vi "CRYGet LoadFileName.vi"(4 "pattern label":string, 5 "ButtonName":string="OK", 6 "pattern (all files)":string="*.cre", 7 "TitleName":string="Open", 8 "error in":errorcluster, 9 "Category Name":string="cre", 10 "default name":string, 11 "Start path":path) -> (0 "error out":errorcluster, 1 "stripped path":path, 2 "Which Button?":T1(ring), 3 "Path":path)   [LabVIEW 2013]
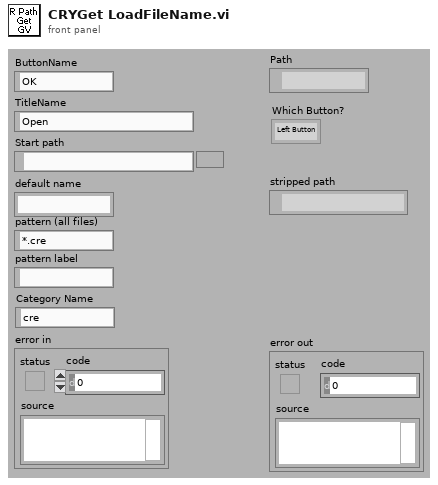
[diagram p1: front panel]
types:
  T1 = enum16{"Left Button", "Center Button", "Right Button", "Window Close"}
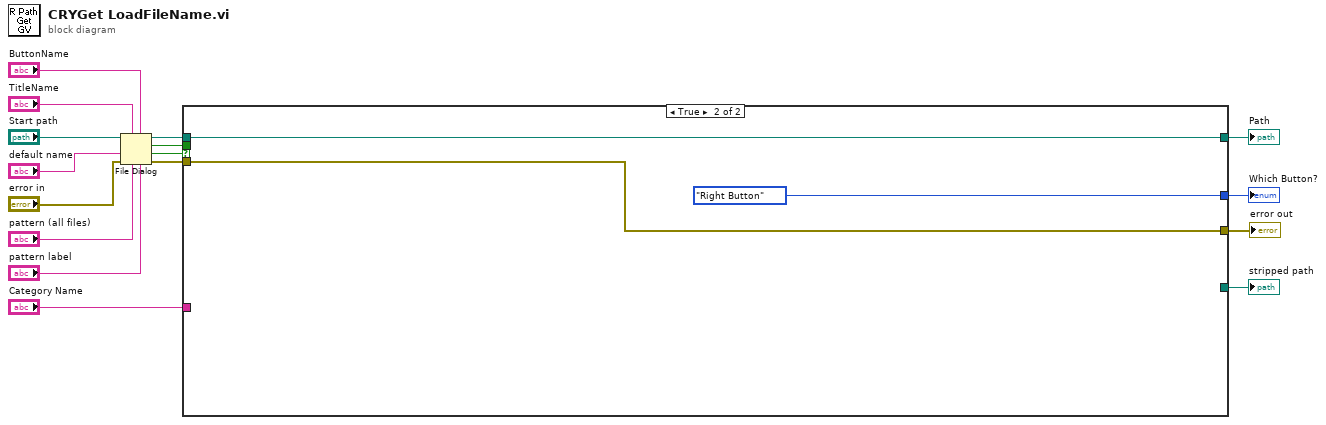
[diagram p0: block diagram]
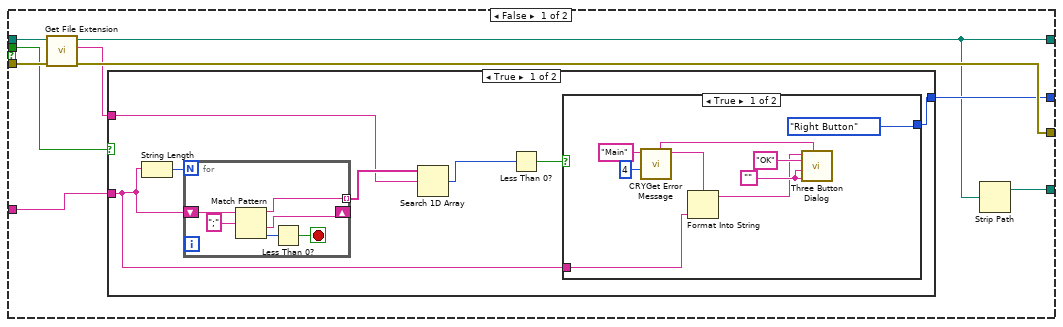
[diagram p2: hidden frame]
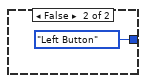
[diagram p3: hidden frame]
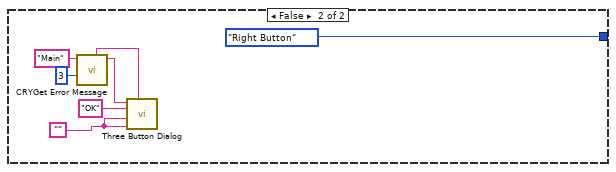
[diagram p4: hidden frame]
diagram:
  n1 = File Dialog(4:"pattern label", 5:"ButtonName", 6:"pattern (all files)", 7:"TitleName", 8:"error in", 9:"default name", 11:"Start path") -> (0:w6:errorcluster, 1:w12:bool, 2:w2:bool, 3:w14:path)
  n2 = case shown="True" w12 {
    tunnel: w14 -> [w25 w58]
    tunnel: "Category Name" -> [w21 _]
    tunnel: [w18 w58] -> w7
    tunnel: w6 -> [w24 w56]
    tunnel: [w23 w56] -> w5
    tunnel: [w20 T1."Right Button" ("Which Button?")] -> w3
    tunnel: w2 -> [w22 _]
    tunnel: [w17 _] -> w1
    frame False {
      n3 = call <vilib>:"Get File Extension.vi"("error in (no error)"=w24, "file"=w25) -> ("error out"=w23:errorcluster, "lowercase file extension"=w19:string, "dup file"=w18:path)  [unwired: 7 out]
      n4 = case shown="True" w22 {
        tunnel: w21 -> [w29 _]
        tunnel: [w32 T1."Right Button" ("Which Button?")] -> w20
        tunnel: w19 -> [w27 _]
        frame True {
          n5 = String Length(string=w29) -> (length=w30:i32)
          n6 = for {
            N: w30 -> [_]
            tunnel: [w37] -> w28 mode=indexing
            shift-right: [w36] -> _
            shift-left: w29 -> [w35]
            stop <- w33 stop-if-true
            n7 = Match Pattern(string=w35, regular expression=";" ("search string/char (-)")) -> (before substring=w37:string, after substring=w36:string, offset past match=w34:i32)  [unwired: 2 out]
            n8 = Less Than 0?(x=w34) -> (x < 0?=w33:bool)
          }
          n9 = Search 1D Array(1D array=w28, element=w27) -> (index of element=w26:i32)  [unwired: 1 out]
          n10 = Less Than 0?(x=w26) -> (x < 0?=w31:bool)
          n11 = case shown="True" w31 {
            tunnel: [T1."Right Button" ("Which Button?") T1."Left Button" ("Which Button?")] -> w32
            tunnel: w29 -> [w42 _]
            frame True {
              w45 = ""
              n12 = call "CRYGet Error Message.vi"("Error No"=4, "Kind"="Main") -> ("Message"=w41:string, "Window Title"=w39:string)  [unwired: 4 in, 4 out]
              n13 = Format Into String(format string=w41, w42) -> (resulting string=w40:string)  [unwired: 2 in, 1 out]
              n14 = call <vilib>:"Three Button Dialog.vi"("Window Title (\"\")"=w39, "Right Button Text (\"Cancel\")"=w45, "Center Button Text (\"No\")"=w45, "Left Button Text (\"Yes\")"="OK" ("Left Button Text (\"Yes\")"), "message"=w40) -> ()  [unwired: 7 out]
            }
            frame False {
            }
          }
        }
        frame False {
          w54 = ""
          n15 = call "CRYGet Error Message.vi"("Error No"=3, "Kind"="Main") -> ("Message"=w50:string, "Window Title"=w49:string)  [unwired: 4 in, 4 out]
          n16 = call <vilib>:"Three Button Dialog.vi"("Window Title (\"\")"=w49, "Right Button Text (\"Cancel\")"=w54, "Center Button Text (\"No\")"=w54, "Left Button Text (\"Yes\")"="OK" ("Left Button Text (\"Yes\")"), "message"=w50) -> ()  [unwired: 7 out]
        }
      }
      n17 = Strip Path(path=w18) -> (stripped path=w17:path)  [unwired: 1 out]
    }
    frame True {
    }
  }
  "Path" <- w7
  "error out" <- w5
  "Which Button?" <- w3
  "stripped path" <- w1
